vi "Create Clean Task.vi"(8 "error in (no error)":errorcluster, 11 "Task Name":string) -> (0 "error out":errorcluster, 3 "task out":refnum<k21>)   [LabVIEW 2019, in "4322.lvlib" / "4322.lvclass"]
uses:
  Library/4322.lvclass
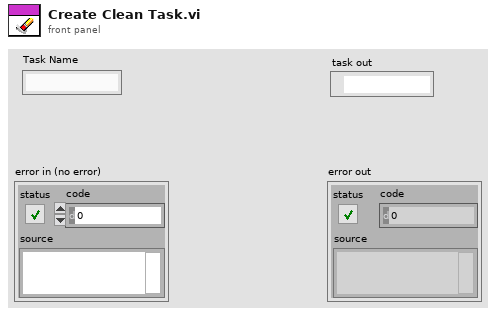
[diagram p1: front panel]
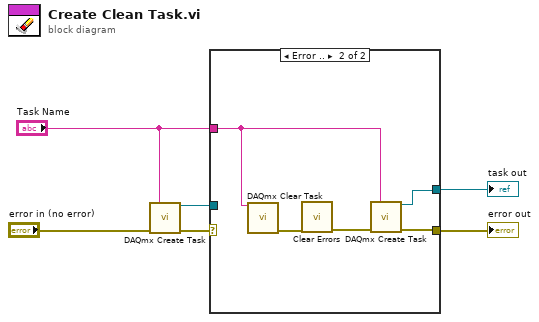
[diagram p0: block diagram]
diagram:
  n1 = call <vilib>:"DAQmx Create Task.vi"("new task name"="Task Name", "error in"="error in (no error)") -> ("task out"=w3:refnum<k21>, "error out"=w5:errorcluster)  [unwired: 12 in]
  n2 = case shown="Error .." w5 {
    selector: w5 -> [w8 _]
    tunnel: [w8 w11] -> w4
    tunnel: w3 -> [w7 _]
    tunnel: "Task Name" -> [_ w9]
    tunnel: [w7 w10] -> w2
    frame No Error {
    }
    frame Error {
      n3 = call <vilib>:"DAQmx Clear Task.vi"("task in"=w9) -> ("error out"=w13:errorcluster)  [unwired: 14 in]
      n4 = call <vilib>:"Clear Errors.vi"("error in (no error)"=w13) -> ("error out"=w12:errorcluster)  [unwired: 5 in, 1 out]
      n5 = call <vilib>:"DAQmx Create Task.vi"("new task name"=w9, "error in"=w12) -> ("task out"=w10:refnum<k21>, "error out"=w11:errorcluster)  [unwired: 12 in]
    }
  }
  "error out" <- w4
  "task out" <- w2
